vi "Format Variant into String Advance.vi"(6 "include Variant Attributes(F)":bool, 8 "error in (no error)":errorcluster, 11 "Variant":variant) -> (0 "error out":errorcluster, 2 "Type Descriptor Enumeration":T1 format="%.0x", 3 "Data":string)   [LabVIEW 2017]
uses:
  <userlib>/_OpenG.lib/lvdata/lvdata.llb/Type Descriptor Enumeration__ogtk.ctl
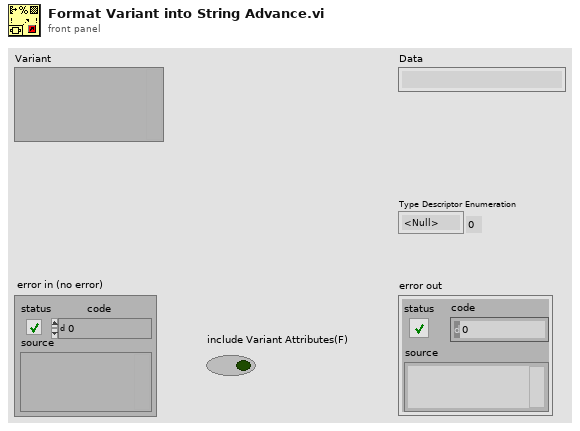
[diagram p1: front panel]
types:
  T1 = typedef "Type Descriptor Enumeration__ogtk.ctl" = enum8{"<Null>", "I8", "I16", "I32", "I64", "U8", "U16", "U32", "U64", "SGL", "DBL", "EXT", "CSG", "CDB", "CXT", "0x0F", "0x10", "0x11", "0x12", "0x13", "0x14", "Enum U8", "Enum U16", "Enum U32", "Enum U64", "SGL PQ", "DBL PQ", "EXT PQ", "CSG PQ", "CDB PQ", "CXT PQ", "0x1F", "0x20", "Boolean", "0x22", "0x23", "0x24", "0x25", "0x26", "0x27", "0x28", "0x29", "0x2A", "0x2B", "0x2C", "0x2D", "0x2E", "0x2F", "String", "0x31", "Path", "Pict", "0x34", "0x35", "0x36", "DAQ", "0x38", "0x39", "0x3A", "0x3B", "0x3C", "0x3D", "0x3E", "0x3F", "Array", "0x41", "0x42", "0x43", "0x44", "0x45", "0x46", "0x47", "0x48", "0x49", "0x4A", "0x4B", "0x4C", "0x4D", "0x4E", "0x4F", "Cluster", "0x51", "0x52", "Variant", "Waveform", "0x55", "0x56", "0x57", "0x58", "0x59", "0x5A", "0x5B", "0x5C", "0x5D", "0x5E", "0x5F", "0x60", "0x61", "0x62", "0x63", "0x64", "0x65", "0x66", "0x67", "0x68", "0x69", "0x6A", "0x6B", "0x6C", "0x6D", "0x6E", "0x6F", "Refnum"}
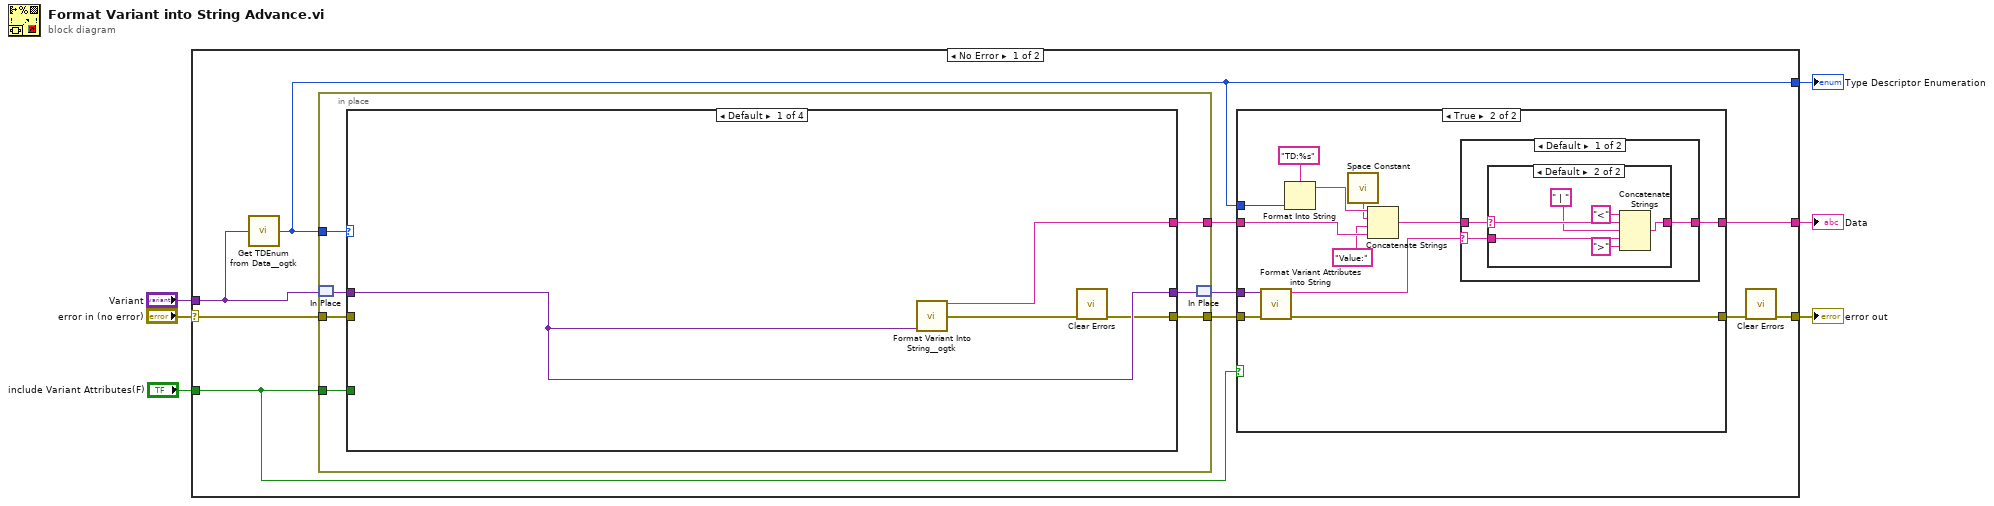
[diagram p0: block diagram]
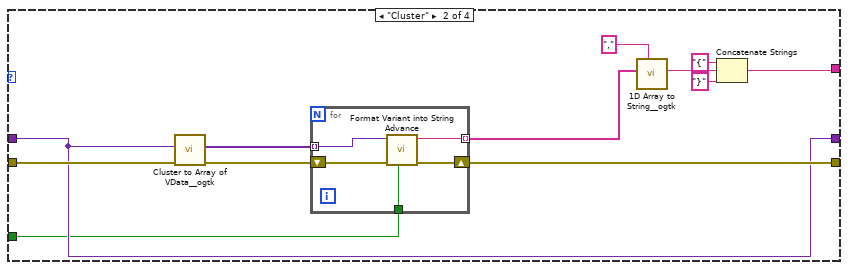
[diagram p5: hidden frame]
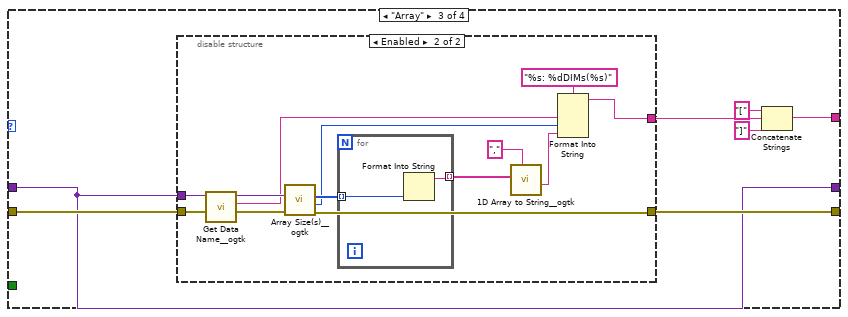
[diagram p6: hidden frame]
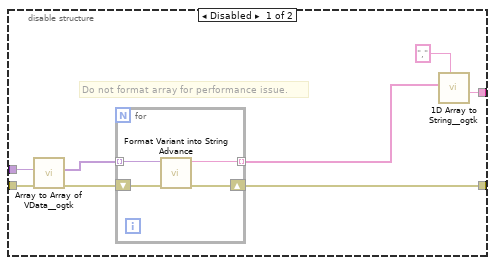
[diagram p7: hidden frame]
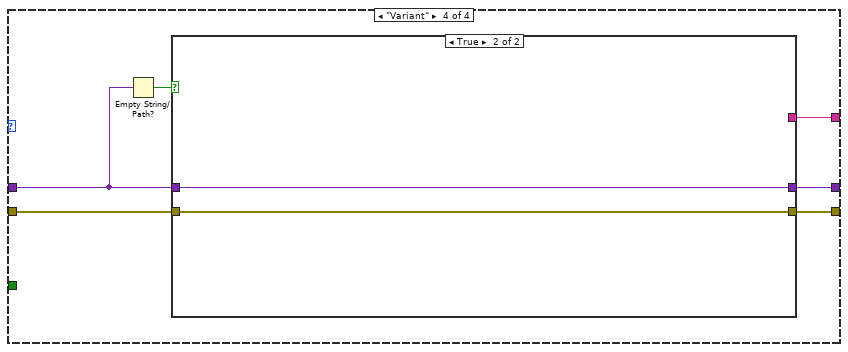
[diagram p8: hidden frame]
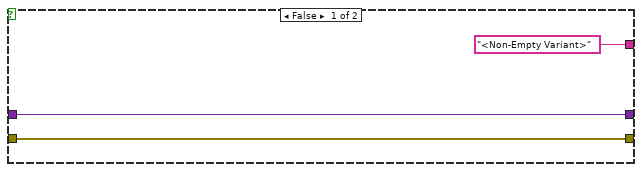
[diagram p9: hidden frame]
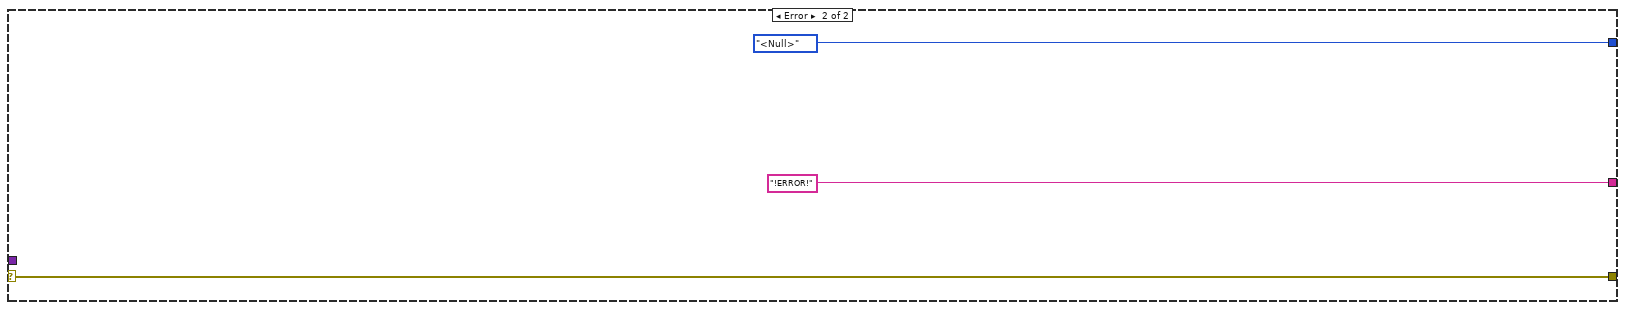
[diagram p10: hidden frame]
diagram:
  n1 = case shown="No Error" "error in (no error)" {
    selector: "error in (no error)" -> [w16 w117]
    tunnel: [w11 "!ERROR!" ("Output String")] -> w6
    tunnel: [w15 w117] -> w4
    tunnel: "Variant" -> [w10 _]
    tunnel: [w7 Type_Descriptor_Enumeration__ogtk."<Null>" ("Type Descriptor Enumeration")] -> w2
    tunnel: "include Variant Attributes(F)" -> [w8 _]
    frame No Error {
      n2 = call <userlib>:"Get TDEnum from Data__ogtk.vi"("Data"=w10) -> ("Type Descriptor Enumeration"=w7:T1)  [unwired: 4 in]
      n3 = in-place {
        in-place-border: w16 -> [w48]
        in-place-border: w7 -> [w47]
        in-place-border: [w46] -> w14
        in-place-border: [w45] -> w12
        in-place-border: w8 -> [w42]
        n4 = in-place-match #1(w10) -> (w44:variant)
        n5 = case shown="Default" w47 {
          tunnel: [w52 w57 w74 w107] -> w45
          tunnel: [w49 w61 w76 w108] -> w46
          tunnel: w44 -> [w50 w54 w70 w104]
          tunnel: w48 -> [_ w58 w71 w109]
          tunnel: [w50 w54 w70 w105] -> w43
          tunnel: w42 -> [_ w53 _ _]
          frame Default {
            n6 = call <userlib>:"Format Variant Into String__ogtk.vi"("Variant"=w50) -> ("Output String"=w52:string, "error out"=w51:errorcluster)  [unwired: 13 in]
            n7 = call <vilib>:"Clear Errors.vi"("error in (no error)"=w51) -> ("error out"=w49:errorcluster)  [unwired: 5 in, 1 out]
          }
          frame "Cluster" {
            n8 = call <userlib>:"Cluster to Array of VData__ogtk.vi"("error in (no error)"=w58, "Cluster"=w54) -> ("error out"=w62:errorcluster, "Array of VData"=w64:variant[])  [unwired: 8 in]
            n9 = for {
              tunnel: w64 -> [w69] mode=indexing
              tunnel: [w68] -> w63 mode=indexing
              shift-right: [w66] -> w61
              shift-left: w62 -> [w67]
              tunnel: w53 -> [w65]
              n10 = call "Format Variant into String Advance.vi"("include Variant Attributes(F)"=w65, "error in (no error)"=w67, "Variant"=w69) -> ("error out"=w66:errorcluster, "Data"=w68:string)  [unwired: 6 in, 1 out]
            }
            n11 = call <userlib>:"1D Array to String__ogtk.vi"("delimiter (Tab)"=",", "Array of Strings"=w63) -> ("delimited string"=w60:string)  [unwired: 9 in]
            n12 = Concatenate Strings("{" ("string"), w60, "}" ("string")) -> (w57:string)
          }
          frame "Array" {
            n13 = disable-structure shown="Enabled" {
              disable-tunnel: w70 -> [w84 w101]
              disable-tunnel: [w80 w93] -> w76
              disable-tunnel: [w79 w89] -> w75
              disable-tunnel: w71 -> [w77 w99]
              frame Disabled {
                # "Do not format array for performance issue."
                n14 = call <userlib>:"Array to Array of VData__ogtk.vi"("error in (no error)"=w77, "MultiD Array"=w84) -> ("error out"=w81:errorcluster, "1D Array of Variants"=w83:variant[])  [unwired: 8 in]
                n15 = for {
                  tunnel: w83 -> [w88] mode=indexing
                  tunnel: [w87] -> w82 mode=indexing
                  shift-right: [w85] -> w80
                  shift-left: w81 -> [w86]
                  n16 = call "Format Variant into String Advance.vi"("error in (no error)"=w86, "Variant"=w88) -> ("error out"=w85:errorcluster, "Data"=w87:string)  [unwired: 7 in, 1 out]
                }
                n17 = call <userlib>:"1D Array to String__ogtk.vi"("delimiter (Tab)"=",", "Array of Strings"=w82) -> ("delimited string"=w79:string)  [unwired: 9 in]
              }
              frame Enabled {
                n18 = call <userlib>:"Get Data Name__ogtk.vi"("error in (no error)"=w99, "Data"=w101) -> ("error out"=w98:errorcluster, "Data Name"=w95:string, "Data dup"=w100:variant)  [unwired: 7 in]
                n19 = call <userlib>:"Array Size(s)__ogtk.vi"("error in (no error)"=w98, "Array"=w100) -> ("error out"=w93:errorcluster, "N dims"=w94:u32, "Size(s)"=w96:u32[])  [unwired: 7 in]
                n20 = for {
                  tunnel: w96 -> [w103] mode=indexing
                  tunnel: [w102] -> w91 mode=indexing
                  n21 = Format Into String(w103) -> (resulting string=w102:string)  [unwired: 3 in, 1 out]
                }
                n22 = call <userlib>:"1D Array to String__ogtk.vi"("delimiter (Tab)"=",", "Array of Strings"=w91) -> ("delimited string"=w90:string)  [unwired: 9 in]
                n23 = Format Into String(format string="%s: %dDIMs(%s)", w95, w94, w90) -> (resulting string=w89:string)  [unwired: 2 in, 1 out]
              }
            }
            n24 = Concatenate Strings("[" ("string"), w75, "]" ("string")) -> (w74:string)
          }
          frame "Variant" {
            n25 = Empty String/Path?(string/path=w104) -> (empty?=w106:bool)
            n26 = case shown="True" w106 {
              tunnel: w109 -> [w111 w114]
              tunnel: [w111 w114] -> w108
              tunnel: ["<Non-Empty Variant>" ("Output String") _] -> w107
              tunnel: [w110 w113] -> w105
              tunnel: w104 -> [w110 w113]
              frame False {
              }
              frame True {
              }
            }
          }
        }
        n27 = in-place-match #1(w43) -> (w9:variant)
      }
      n28 = case shown="True" w8 {
        tunnel: w14 -> [w17 w30]
        tunnel: [w17 w29] -> w13
        tunnel: w12 -> [w18 w22]
        tunnel: [w18 w28] -> w11
        tunnel: w9 -> [_ w26]
        tunnel: w7 -> [_ w25]
        frame False {
        }
        frame True {
          n29 = call "Format Variant Attributes into String.vi"("error in (no error)"=w30, "Variant"=w26) -> ("error out"=w29:errorcluster, "Data"=w27:string)  [unwired: 8 in]
          n30 = Format Into String(format string="TD:%s", w25) -> (resulting string=w21:string)  [unwired: 2 in, 1 out]
          n31 = call <vilib>:"Space Constant.vi"() -> ("String"=w19:string)
          n32 = Concatenate Strings(w21, w19, "Value:" ("string"), w22) -> (w23:string)
          n33 = case shown="Default" w27 {
            selector: w27 -> [w31 _]
            tunnel: w23 -> [w33 w41]
            tunnel: [w32 w41] -> w28
            frame Default {
              n34 = case shown="Default" w33 {
                selector: w33 -> [_ w40]
                tunnel: [w34 w39] -> w32
                tunnel: w31 -> [w34 w38]
                frame "" {
                }
                frame Default {
                  n35 = Concatenate Strings("<" ("string"), w40, " | " ("string"), w38, ">" ("string")) -> (w39:string)
                }
              }
            }
            frame "" {
            }
          }
        }
      }
      n36 = call <vilib>:"Clear Errors.vi"("error in (no error)"=w13) -> ("error out"=w15:errorcluster)  [unwired: 5 in, 1 out]
    }
    frame Error {
    }
  }
  "Data" <- w6
  "error out" <- w4
  "Type Descriptor Enumeration" <- w2
